vi "Update Layout.vi"(6 "Sync Response":refnum<notifier>, 8 "error in (no error)":errorcluster, 10 "Synced":bool, 11 "2DArrayManager in":refnum<class "2DArrayManager.lvclass">) -> (0 "error out":errorcluster, 3 "2DArrayManager out":refnum<class "2DArrayManager.lvclass">)   [LabVIEW 2020, in "OOPanel.lvlib" / "2DArrayManager.lvclass"]
uses:
  2DArrayManager.lvclass
  2DArrayManager.lvclass/2DArrayManager.ctl
  ArrayPanel/ArrayPanel.lvclass
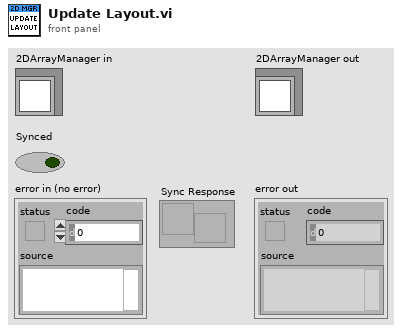
[diagram p1: front panel]
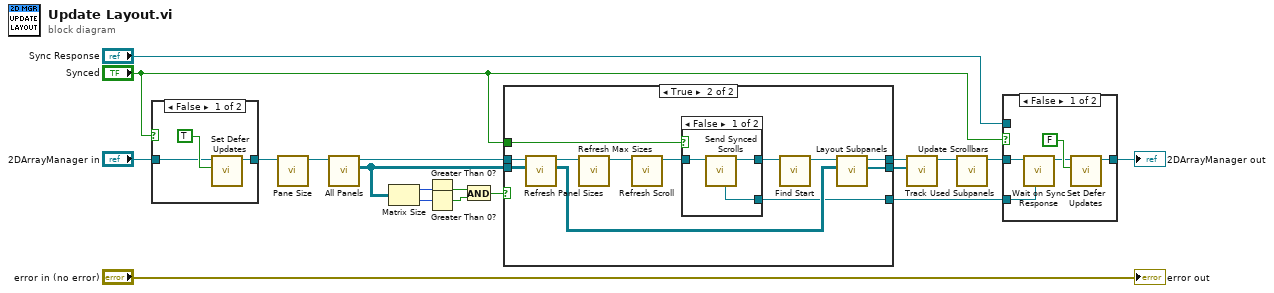
[diagram p0: block diagram]
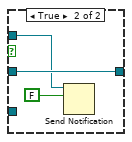
[diagram p5: hidden frame]
diagram:
  n1 = case shown="False" "Synced" {
    tunnel: "2DArrayManager in" -> [w21 w23]
    tunnel: [w20 w23] -> w17
    frame False {
      n2 = call "Set Defer Updates.vi"("Defer Updates"=TRUE, "2DArrayManager in"=w21) -> ("2DArrayManager out"=w20:refnum<class "2DArrayManager.lvclass">)  [unwired: 8 in, 1 out]
    }
    frame True {
    }
  }
  n3 = call "Pane Size.vi"("2DArrayManager in"=w17) -> ("2DArrayManager out"=w8:refnum<class "2DArrayManager.lvclass">)  [unwired: 9 in, 1 out]
  n4 = call "All Panels.vi"("2DArrayManager in"=w8) -> ("Panels"=w10:refnum<class "ArrayPanel.lvclass">[][], "2DArrayManager out"=w11:refnum<class "2DArrayManager.lvclass">)  [unwired: 8 in, 1 out]
  n5 = Matrix Size(0:w10) -> (1:w16:i32, 2:w15:i32)
  n6 = Greater Than 0?(x=w16) -> (x > 0?=w14:bool)
  n7 = Greater Than 0?(x=w15) -> (x > 0?=w13:bool)
  n8 = And(x=w14, y=w13) -> (x .and. y?=w12:bool)
  n9 = case shown="True" w12 {
    tunnel: w11 -> [w24 w36]
    tunnel: w10 -> [_ w35]
    tunnel: [w24 w30] -> w3
    tunnel: "Synced" -> [_ w29]
    tunnel: [_ w26] -> w5
    tunnel: [_ w25] -> w1
    frame False {
    }
    frame True {
      n10 = call "Refresh Panel Sizes.vi"("Panels in"=w35, "2DArrayManager in"=w36) -> ("Panels"=w31:refnum<class "ArrayPanel.lvclass">[][], "2DArrayManager out"=w34:refnum<class "2DArrayManager.lvclass">)  [unwired: 7 in, 1 out]
      n11 = call "Refresh Max Sizes.vi"("2DArrayManager in"=w34) -> ("2DArrayManager out"=w33:refnum<class "2DArrayManager.lvclass">)  [unwired: 9 in, 1 out]
      n12 = call "Refresh Scroll.vi"("2DArrayManager in"=w33) -> ("2DArrayManager out"=w28:refnum<class "2DArrayManager.lvclass">)  [unwired: 9 in, 1 out]
      n13 = case shown="False" w29 {
        tunnel: w28 -> [w39 w40]
        tunnel: [w38 w40] -> w27
        tunnel: [w37 _] -> w26
        frame False {
          n14 = call "Send Synced Scrolls.vi"("2DArrayManager in"=w39) -> ("2DArrayManager out"=w38:refnum<class "2DArrayManager.lvclass">, "Sync Response"=w37:refnum<notifier>)  [unwired: 8 in, 1 out]
        }
        frame True {
        }
      }
      n15 = call "Find Start.vi"("2DArrayManager in"=w27) -> ("2DArrayManager out"=w32:refnum<class "2DArrayManager.lvclass">)  [unwired: 9 in, 1 out]
      n16 = call "Layout Subpanels.vi"("Panels in"=w31, "2DArrayManager in"=w32) -> ("Used SubPanels"=w25:refnum<vi>[], "2DArrayManager out"=w30:refnum<class "2DArrayManager.lvclass">)  [unwired: 6 in, 2 out]
    }
  }
  n17 = call "Track Used Subpanels.vi"("Used SubPanels"=w1, "2DArrayManager in"=w3) -> ("2DArrayManager out"=w2:refnum<class "2DArrayManager.lvclass">)  [unwired: 8 in, 1 out]
  n18 = call "Update Scrollbars.vi"("2DArrayManager in"=w2) -> ("2DArrayManager out"=w7:refnum<class "2DArrayManager.lvclass">)  [unwired: 9 in, 1 out]
  n19 = case shown="False" "Synced" {
    tunnel: [w45 w48] -> w9
    tunnel: w7 -> [w43 w48]
    tunnel: w5 -> [w41 _]
    tunnel: "Sync Response" -> [_ w46]
    frame False {
      n20 = call "Wait on Sync Response.vi"("Sync Response"=w41, "2DArrayManager in"=w43) -> ("2DArrayManager out"=w42:refnum<class "2DArrayManager.lvclass">)  [unwired: 8 in, 1 out]
      n21 = call "Set Defer Updates.vi"("Defer Updates"=FALSE, "2DArrayManager in"=w42) -> ("2DArrayManager out"=w45:refnum<class "2DArrayManager.lvclass">)  [unwired: 8 in, 1 out]
    }
    frame True {
      n22 = Send Notification(notification=FALSE, notifier=w46) -> ()  [unwired: 1 in, 2 out]
    }
  }
  "2DArrayManager out" <- w9
  "error out" <- "error in (no error)"
